vi "CalcAeroTq.vi"(4 "GenSpeed":dbl, 5 "WindSpeed":dbl, 6 "Xi":dbl, 7 "SimulationConst":T1={"nGear"=0.0, "rotorRadius"=0.0, "numBlades"=1, "scaleFactor"=3.0, "roscoInitMinSpeed_rad_s"=0.0, "roscoInitMinTorqueFS_Nm"=0.0, "beckhoff16bit"=0.5, "beckhoff24BitExt"=0, "BX824Bit"=0, "rotorTorqueScale_Nm_V"=0.5, "rotorTorqueOfst_Nm"=0.5, "rangeEL3104V"=0.5, "nacelleAccELM3604V"=0.5, "nacelleAccScaleX_m_s2_V"=0.5, "nacelleAccOfstX_m_s2"=0.5, "nacelleAccScaleY_m_s2_V"=0.5, "nacelleAccOfstY_m_s2"=0.5, "nacelleAccScaleZ_m_s2_V"=0.5, "nacelleAccOfstZ_m_s2"=0.5, "cyberGearRatio"=0.5, "cyberLinesPerRev"=0.5, "cyberRatedTorque"=0.5, "towerTopForceScale"=0.5, "towerTopTorqueScale"=0.5, "plcSetpointScaling_norm2VFD"=0.5, "towerBotScaleMy_Nm_V"=0.5, "towerBotOfstMy_Nm"=0.5, "towerTopScaleXaxis_N_V"=0.5, "towerTopOfstXaxis_N"=0.5, "towerTopScaleYaxis_N_V"=0.5, "towerTopOfstYaxis_N"=0.5, "pitchFlagOffset_deg"=0.5, "anemWindSpeedScaleU_m_s_m_s"=0.5, "anemWindSpeedOfstU_m_s"=0.5, "anemWindSpeedScaleV_m_s_m_s"=0.5, "anemWindSpeedOfstV_m_s"=0.5, "anemWindSpeedScaleW_m_s_m_s"=0.5, "anemWindSpeedOfstW_m_s"=0.5, "anemWindSpeedScaleTSI1_m_s_V"=0.5, "anemWindSpeedOfstTSI1_m_s"=0.5, "anemWindSpeedScaleTSI2_m_s_V"=0.5, "anemWindSpeedOfstTSI2_m_s"=0.5, "anemWindSpeedScaleXProbeA1C0_m_s"=0.5, "anemWindSpeedScaleXProbeA1C1_m_s"=0.5, "anemWindSpeedScaleXProbeA1C2_m_s"=0.5, "anemWindSpeedScaleXProbeA1C3_m_s"=0.5, "anemWindSpeedScaleXProbeA1C4_m_s"=0.5, "anemWindSpeedOfstXProbeA1_m_s"=0.5, "anemWindSpeedScaleXProbeA2C0_m_s"=0.5, "anemWindSpeedScaleXProbeA2C1_m_s"=0.5, "anemWindSpeedScaleXProbeA2C2_m_s"=0.5, "anemWindSpeedScaleXProbeA2C3_m_s"=0.5, "anemWindSpeedScaleXProbeA2C4_m_s"=0.5, "anemWindSpeedOfstXProbeA2_m_s"=0.5, "anemWindSpeedOfstHw3_m_s"=0.5, "anemWindSpeedScaleHw3_m_s_V"=0.5, "probeAOfstX_mm"=0.5, "probeAOfstY_mm"=0.5, "probeAOfstZ_mm"=0.5, "probeTSIOfstX_mm"=0.5, "probeTSIOfstY_mm"=0.5, "probeTSIOfstZ_mm"=0.5, "probeBOfstX_mm"=0.5, "probeBOfstY_mm"=0.5, "probeBOfstZ_mm"=0.5}, 8 "tsr(Y)":dbl[](array[numeric]), 9 "pitch (X)":dbl[](array[numeric]), 10 "Cp(Z)":dbl[][](array[numeric])) -> (0 "Cp":dbl, 3 "Ta":dbl)   [LabVIEW 2018]
uses:
  <vilib>/gmath/NI_Gmath.lvlib
  <vilib>/gmath/interp.llb/Interpolate 2D (1d xi,yi).vi
  Clusters/SimulationConstants.ctl
panel:
  out "CpArr":dbl[][](array[numeric])
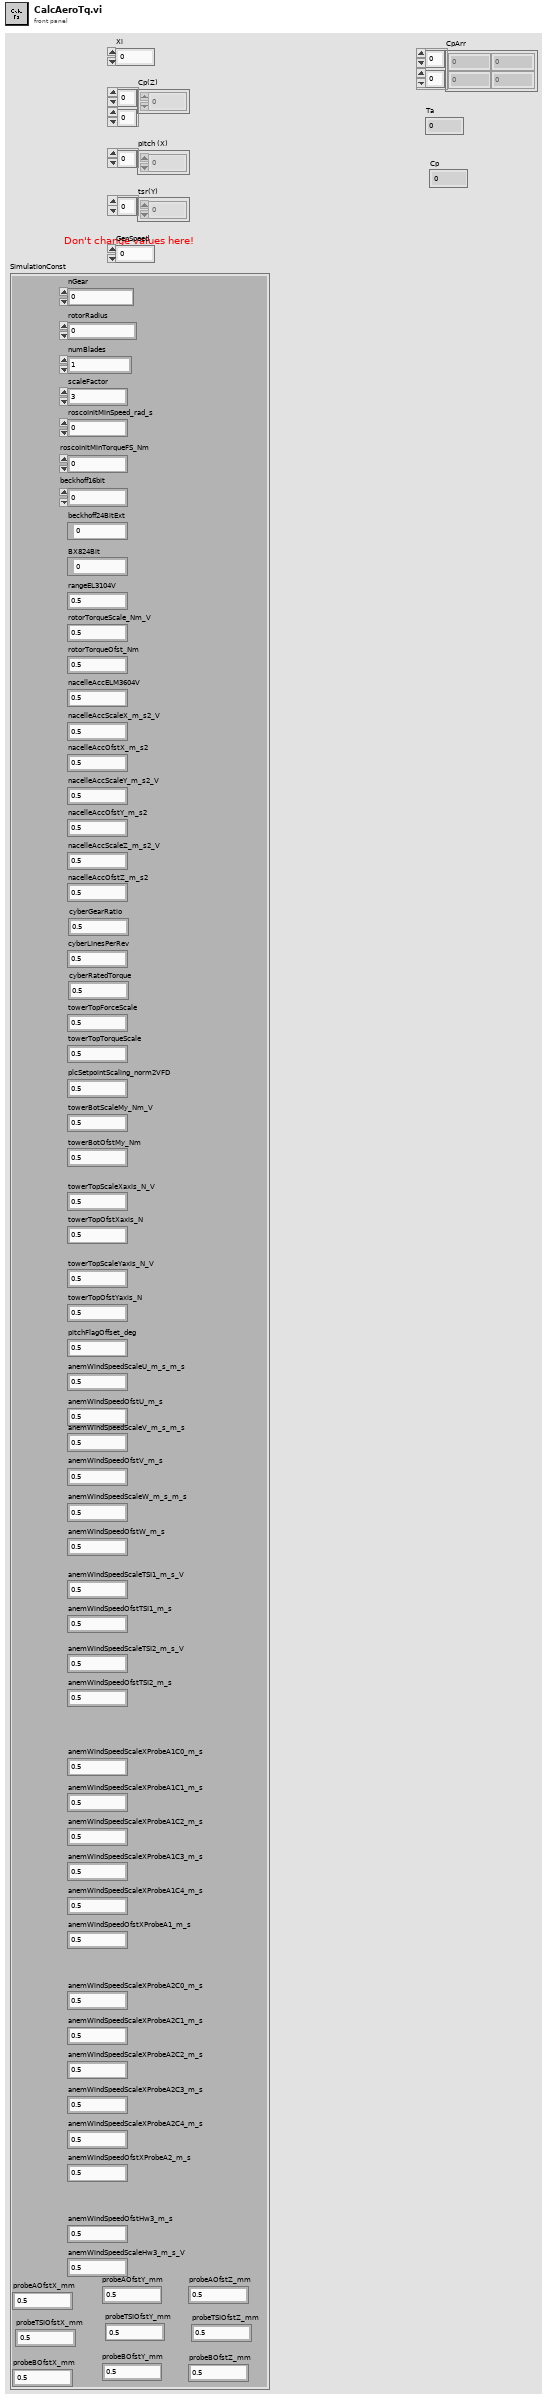
[diagram p1: front panel]
types:
  T1 = typedef "SimulationConstants.ctl" = cluster{"nGear":dbl, "rotorRadius":sgl, "numBlades":i32, "scaleFactor":dbl, "roscoInitMinSpeed_rad_s":dbl, "roscoInitMinTorqueFS_Nm":dbl, "beckhoff16bit":dbl, "beckhoff24BitExt":i32, "BX824Bit":i32, "rotorTorqueScale_Nm_V":dbl, "rotorTorqueOfst_Nm":dbl, "rangeEL3104V":dbl, "nacelleAccELM3604V":dbl, "nacelleAccScaleX_m_s2_V":dbl, "nacelleAccOfstX_m_s2":dbl, "nacelleAccScaleY_m_s2_V":dbl, "nacelleAccOfstY_m_s2":dbl, "nacelleAccScaleZ_m_s2_V":dbl, "nacelleAccOfstZ_m_s2":dbl, "cyberGearRatio":dbl, "cyberLinesPerRev":dbl, "cyberRatedTorque":dbl, "towerTopForceScale":dbl, "towerTopTorqueScale":dbl, "plcSetpointScaling_norm2VFD":dbl, "towerBotScaleMy_Nm_V":dbl, "towerBotOfstMy_Nm":dbl, "towerTopScaleXaxis_N_V":dbl, "towerTopOfstXaxis_N":dbl, "towerTopScaleYaxis_N_V":dbl, "towerTopOfstYaxis_N":dbl, "pitchFlagOffset_deg":dbl, "anemWindSpeedScaleU_m_s_m_s":dbl, "anemWindSpeedOfstU_m_s":dbl, "anemWindSpeedScaleV_m_s_m_s":dbl, "anemWindSpeedOfstV_m_s":dbl, "anemWindSpeedScaleW_m_s_m_s":dbl, "anemWindSpeedOfstW_m_s":dbl, "anemWindSpeedScaleTSI1_m_s_V":dbl, "anemWindSpeedOfstTSI1_m_s":dbl, "anemWindSpeedScaleTSI2_m_s_V":dbl, "anemWindSpeedOfstTSI2_m_s":dbl, "anemWindSpeedScaleXProbeA1C0_m_s":dbl, "anemWindSpeedScaleXProbeA1C1_m_s":dbl, "anemWindSpeedScaleXProbeA1C2_m_s":dbl, "anemWindSpeedScaleXProbeA1C3_m_s":dbl, "anemWindSpeedScaleXProbeA1C4_m_s":dbl, "anemWindSpeedOfstXProbeA1_m_s":dbl, "anemWindSpeedScaleXProbeA2C0_m_s":dbl, "anemWindSpeedScaleXProbeA2C1_m_s":dbl, "anemWindSpeedScaleXProbeA2C2_m_s":dbl, "anemWindSpeedScaleXProbeA2C3_m_s":dbl, "anemWindSpeedScaleXProbeA2C4_m_s":dbl, "anemWindSpeedOfstXProbeA2_m_s":dbl, "anemWindSpeedOfstHw3_m_s":dbl, "anemWindSpeedScaleHw3_m_s_V":dbl, "probeAOfstX_mm":dbl, "probeAOfstY_mm":dbl, "probeAOfstZ_mm":dbl, "probeTSIOfstX_mm":dbl, "probeTSIOfstY_mm":dbl, "probeTSIOfstZ_mm":dbl, "probeBOfstX_mm":dbl, "probeBOfstY_mm":dbl, "probeBOfstZ_mm":dbl}
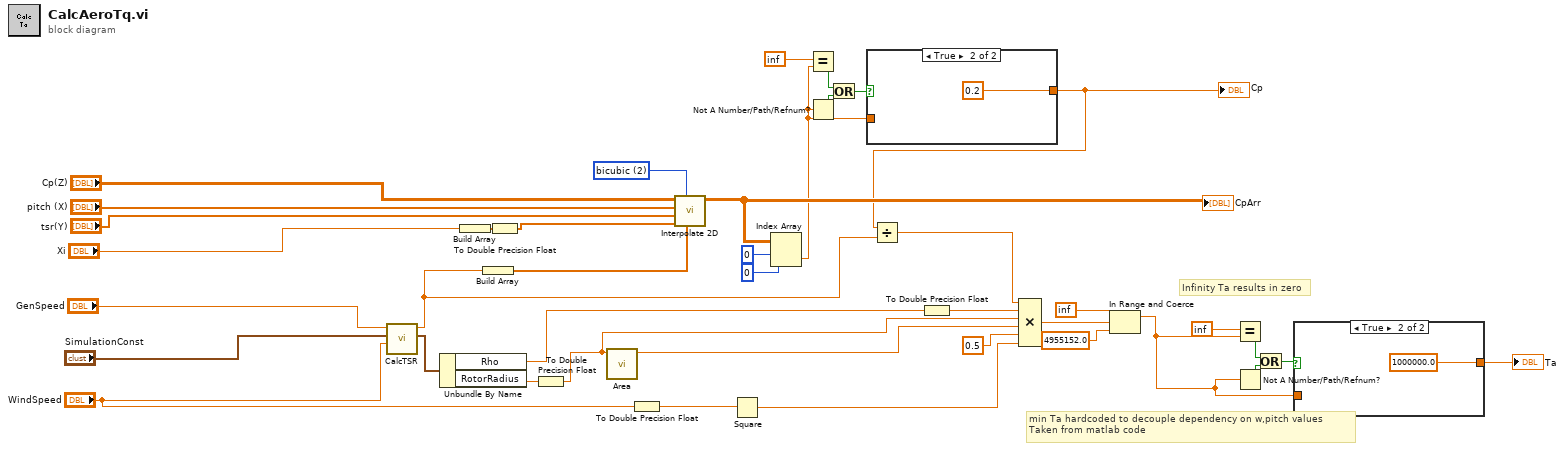
[diagram p0: block diagram]
diagram:
  w16 = 2 items=["nearest", "bilinear", "bicubic", "bicubic spline"] ("method")
  # "min Ta hardcoded to decouple dependency on w,pitch values\nTaken from matlab code"
  # "Infinity Ta results in zero"
  n1 = call "CalcTSR.vi"("WindSpeed"="WindSpeed", "SimulationConst"="SimulationConst", "GenSpeed"="GenSpeed") -> ("SimulationConst Out"=w34:T1, "TSR"=w30:dbl)  [unwired: 7 in]
  n2 = Unbundle By Name(w34) -> ("Rho"=w28:dbl, "RotorRadius"=w29:sgl)
  n3 = Build Array("Xi") -> (w21:dbl[])
  n4 = Build Array(w30) -> (w23:dbl[])
  n5 = To Double Precision Float(number=w21) -> (double precision float=w35:dbl[])
  n6 = To Double Precision Float(number=w29) -> (double precision float=w39:dbl)
  n7 = call "Area.vi"("Numeric in"=w39) -> ("Numeric out"=w40:dbl)  [unwired: 10 in]
  n8 = To Double Precision Float(number="WindSpeed") -> (double precision float=w36:dbl)
  n9 = call-poly <vilib>:"Interpolate 2D.vi"("yi"=w23, "method"=w16, "xi"=w35, "Y"="tsr(Y)", "X"="pitch (X)", "Z"="Cp(Z)") -> ("zi"=w24:dbl[][])  [unwired: 2 in, 3 out]
  "CpArr" <- w24
  n10 = Square(x=w36) -> (x^2=w31:dbl)
  n11 = Index Array(array=w24, index (row)=0, index (col)=0 ("disabled index (col)")) -> (element=w14:dbl)
  n12 = Equal?(x=inf, y=w14) -> (x = y?=w13:bool)
  n13 = Not A Number/Path/Refnum?(number/path/refnum=w14) -> (NaN/Path/Refnum?=w12:bool)
  n14 = Or(x=w13, y=w12) -> (x .or. y?=w11:bool)
  n15 = case shown="True" w11 {
    tunnel: [w41 0.2] -> w1
    tunnel: w14 -> [w41 _]
    frame False {
    }
    frame True {
    }
  }
  "Cp" <- w1
  n16 = Divide(x=w1, y=w30) -> (x/y=w38:dbl)
  n17 = To Double Precision Float(number=w28) -> (double precision float=w32:dbl)
  n18 = Compound Arithmetic op=MULTIPLY(w38, w32, w39, w40, 0.5, w31) -> (w4:dbl)
  n19 = In Range and Coerce(upper limit=inf, x=w4, lower limit=4955152.0) -> (coerced(x)=w2:dbl)  [unwired: 1 out]
  n20 = Equal?(x=inf, y=w2) -> (x = y?=w9:bool)
  n21 = Not A Number/Path/Refnum?(number/path/refnum=w2) -> (NaN/Path/Refnum?=w8:bool)
  n22 = Or(x=w9, y=w8) -> (x .or. y?=w7:bool)
  n23 = case shown="True" w7 {
    tunnel: [w43 1000000.0] -> w6
    tunnel: w2 -> [w43 _]
    frame False {
    }
    frame True {
    }
  }
  "Ta" <- w6
